vi "add_visa_in_control.vi"(8 "error in (no error)":errorcluster, 10 "BD Position":cluster{"Left":i32, "Top":i32}, 11 "VI Ref In":refnum<vi>) -> (0 "error out":errorcluster, 2 "Control Ref Out":refnum<vi>, 3 "VI Ref Out":refnum<vi>)   [LabVIEW 2018]
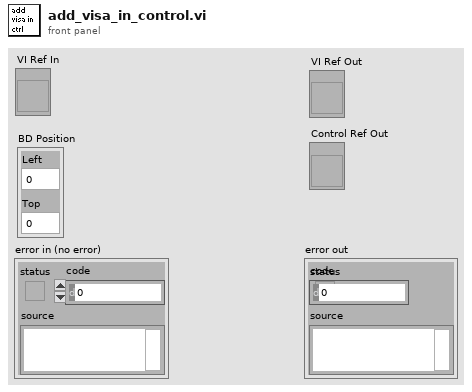
[diagram p1: front panel]
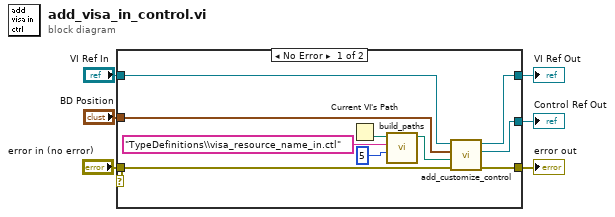
[diagram p0: block diagram]
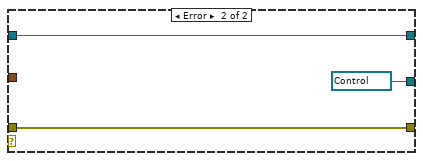
[diagram p2: hidden frame]
diagram:
  n1 = case shown="No Error" "error in (no error)" {
    tunnel: "VI Ref In" -> [w11 w17]
    tunnel: "error in (no error)" -> [w10 w19]
    tunnel: [w8 refnum<vi> refnum ("Ctl Refnum")] -> w5
    tunnel: [w7 w19] -> w4
    tunnel: [w12 w17] -> w2
    tunnel: "BD Position" -> [w9 _]
    frame No Error {
      n2 = Current VI's Path() -> (path=w16:path)
      n3 = call "build_paths.vi"("Numeric"=5, "name or relative path"="TypeDefinitions\\visa_resource_name_in.ctl", "path"=w16) -> ("appended path"=w13:path)  [unwired: 6 out]
      n4 = call "add_customize_control.vi"("error in"=w10, "Control Path"=w13, "Control Position on BD"=w9, "VI Ref In"=w11) -> ("error out"=w7:errorcluster, "Ctl Refnum"=w8:refnum<vi>, "VI Ref Out"=w12:refnum<vi>)  [unwired: 5 out]
    }
    frame Error {
    }
  }
  "VI Ref Out" <- w2
  "Control Ref Out" <- w5
  "error out" <- w4
